vi "Element Init.vi"(7 "VolatusAPI":refnum<class "VolatusAPI.lvclass">, 8 "error in (no error)":errorcluster, 10 "JSON":string, 11 "GaugeIndicator in":refnum<class "GaugeIndicator.lvclass">) -> (0 "error out":errorcluster, 3 "GaugeIndicator out":refnum<class "GaugeIndicator.lvclass">)   [LabVIEW 2023, in "VolatusGUIElements.lvlib" / "GaugeIndicator.lvclass"]
uses:
  GaugeIndicator.lvclass
  Volatus/VolatusAPI/VolatusAPI.lvclass
  GaugeIndicator.lvclass/GaugeIndicator.ctl
  lv-cdm/CDM-Config/Config-JSON/Config-JSON.lvclass
  lv-cdm/CDM-Config/Config Manager/Config Manager.lvclass
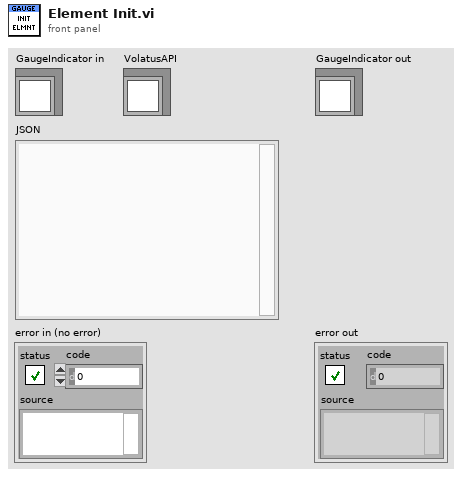
[diagram p1: front panel]
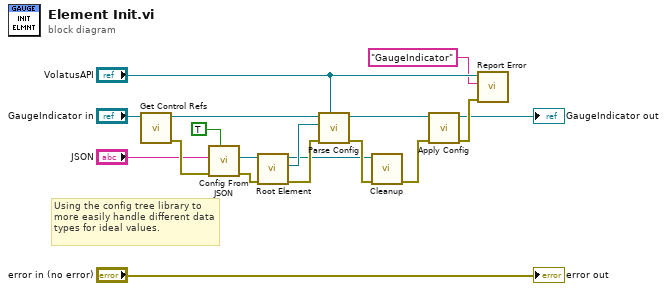
[diagram p0: block diagram]
diagram:
  # "Using the config tree library to more easily handle different data types for ideal values."
  n1 = call "Get Control Refs.vi"("GaugeIndicator in"="GaugeIndicator in") -> ("error out"=w16:errorcluster, "GaugeIndicator out"=w13:refnum<class "GaugeIndicator.lvclass">)  [unwired: 9 in]
  n2 = call "Config From JSON.vi"("Mutable (F)"=TRUE, "error in (no error)"=w16, "JSON"="JSON") -> ("error out"=w10:errorcluster, "Config"=w11:refnum<class "Config Manager.lvclass">)  [unwired: 7 in]
  n3 = call "Root Element.vi"("error in (no error)"=w10, "Config Manager in"=w11) -> ("error out"=w7:errorcluster, "Root Element"=w8:refnum<class "Config Element.lvclass">, "Config Manager out"=w6:refnum<class "Config Manager.lvclass">)  [unwired: 7 in]
  n4 = call "Parse Config.vi"("VolatusAPI"="VolatusAPI", "error in (no error)"=w7, "Config Element"=w8, "GaugeIndicator in"=w13) -> ("error out"=w17:errorcluster, "GaugeIndicator out"=w9:refnum<class "GaugeIndicator.lvclass">)  [unwired: 6 in]
  n5 = call "Cleanup.vi"("error in (no error)"=w17, "Config Manager in"=w6) -> ("error out"=w4:errorcluster)  [unwired: 9 in]
  n6 = call "Apply Config.vi"("error in (no error)"=w4, "GaugeIndicator in"=w9) -> ("error out"=w18:errorcluster, "GaugeIndicator out"=→"GaugeIndicator out":refnum<class "GaugeIndicator.lvclass">)  [unwired: 8 in]
  n7 = call "Report Error.vi"("error in (no error)"=w18, "Context"="GaugeIndicator", "VolatusAPI in"="VolatusAPI") -> ()  [unwired: 7 in, 2 out]
  "error out" <- "error in (no error)"
